vi "Sequence.BuildSetup.vi"(8 "error in (no error)":errorcluster, 11 "Sequence":refnum<k24>) -> (0 "error out":errorcluster, 3 "Sequence out":refnum<k24>)   [LabVIEW 2013, in "Simple Sequence Editor.lvlib"]
uses:
  Simple Sequence Editor.lvlib
  NationalInstruments.VeriStand.RealTimeSequenceDefinitionApi
  Constants.vi
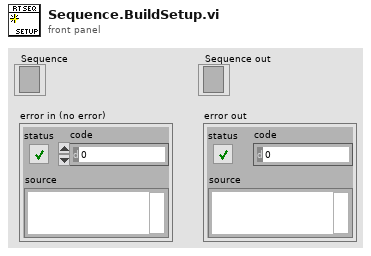
[diagram p1: front panel]
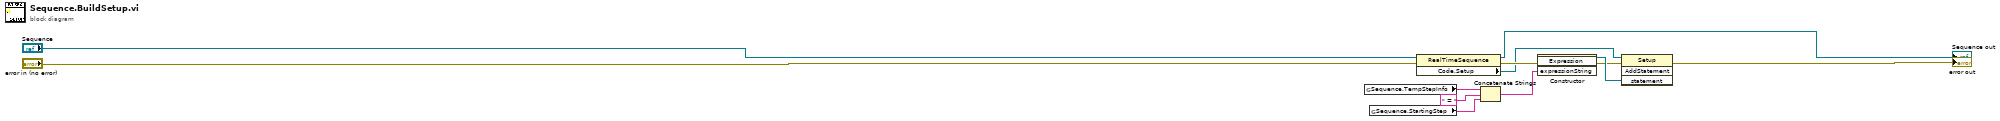
[diagram p0: block diagram]
diagram:
  n1 = global read "Constants.vi" "Sequence.TempStepInfo"() -> (w9:string)
  n2 = global read "Constants.vi" "Sequence.StartingStep"() -> (w10:string)
  n3 = property class="RealTimeSequence"(reference="Sequence", error in="error in (no error)") -> (reference out=→"Sequence out":refnum<k24>, error out=w6:errorcluster, "Code.Setup"=w4:refnum<k24>)
  n4 = Concatenate Strings(w9, " = " ("expressionString"), w10) -> (w12:string)
  n5 = constructor class="Expression"(error in=w6, "expressionString"=w12) -> (reference out=w8:refnum<k24>, error out=w5:errorcluster)  [unwired: 2 in, 2 out]
  n6 = invoke class="Setup" method="AddStatement"(reference=w4, error in=w5, "statement"=w8) -> (error out=→"error out":errorcluster)  [unwired: 1 in, 3 out]
